vi "FTW-ERR-StatusOK.vi"(1 "error to check":errorcluster) -> (0 "Status OK?":bool)   [LabVIEW 2015]
panel:
  # "Inputs"
  # "Outputs"
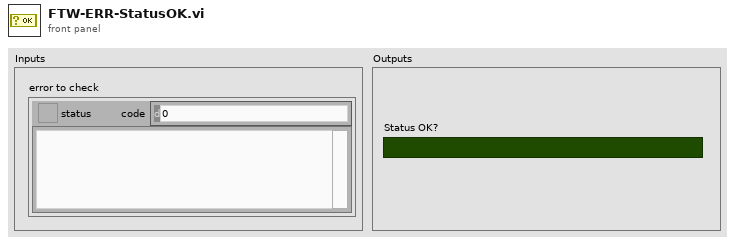
[diagram p1: front panel]
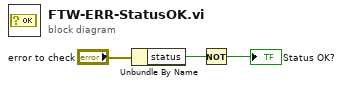
[diagram p0: block diagram]
diagram:
  n1 = Unbundle By Name("error to check") -> ("status"=w2:bool)
  n2 = Not(x=w2) -> (.not. x?=→"Status OK?":bool)
